vi "Teleop.vi"(10 "Match Info":T1={"Autonomous Elapsed Seconds"=0.0, "TeleOp Elapsed Seconds"=0.0, "Disabled Elapsed Seconds"=0.0, "Visited Autonomous"=FALSE, "Visited TeleOp"=FALSE, "Visited Disabled"=FALSE, "Autonomous Settings"={"Autonomous Style"=enum."Independent", "VI Refnum"=refnum}}, 11 "Call Context":T2) -> ()   [LabVIEW 2020]
doc: "This VI is called for each enabled TeleOp packet received from the DS. It is typically used to read from joysticks and other inputs and update I/O or setpoints for timed control loops. It should complete and return within 20 milliseconds or risk missing DS packets."
uses:
  <vilib>/Rock Robotics/WPI/DriverStation/WPI_DriverStationDerivedRobotMode.ctl
  <vilib>/Rock Robotics/WPI/DriverStation/WPI_DriverStationMatch Info.ctl
  <vilib>/Rock Robotics/WPI/Utilities/WPI_GetSetVariantRefNum.vi
  <vilib>/Rock Robotics/Network Tables/NT Write Boolean Array.vi
  <vilib>/Rock Robotics/Network Tables/NT Write Numeric Array.vi
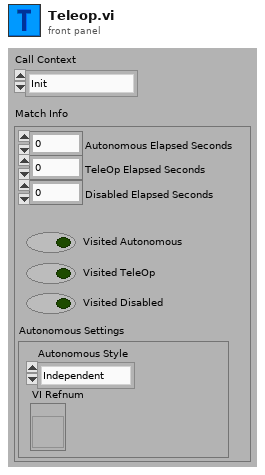
[diagram p1: front panel]
types:
  T1 = typedef "WPI_DriverStationMatch Info.ctl" = cluster{"Autonomous Elapsed Seconds":dbl, "TeleOp Elapsed Seconds":dbl, "Disabled Elapsed Seconds":dbl, "Visited Autonomous":bool, "Visited TeleOp":bool, "Visited Disabled":bool, "Autonomous Settings":cluster{"Autonomous Style":enum16{"Iterative", "Independent"}, "VI Refnum":refnum<vi>}}
  T2 = typedef "WPI_DriverStationDerivedRobotMode.ctl" = enum16{"Init", "Execute", "Stop"}
  T3 = typedef "WPI_JoystickDevRef.ctl" = cluster{"Device":T4}
  T4 = typedef "WPI_JoystickDeviceEnum.ctl" = enum16{"USB 0", "USB 1", "USB 2", "USB 3", "USB 4", "USB 5"}
  T5 = typedef "Command Status Info.ctl" = cluster{"Name":string, "Status":T6, "notifier out":T7}
  T6 = typedef "Completion Status.ctl" = enum16{"Successful", "Aborted", "Incomplete"}
  T7 = typedef "Completion Notifier.ctl" = refnum<notifier>
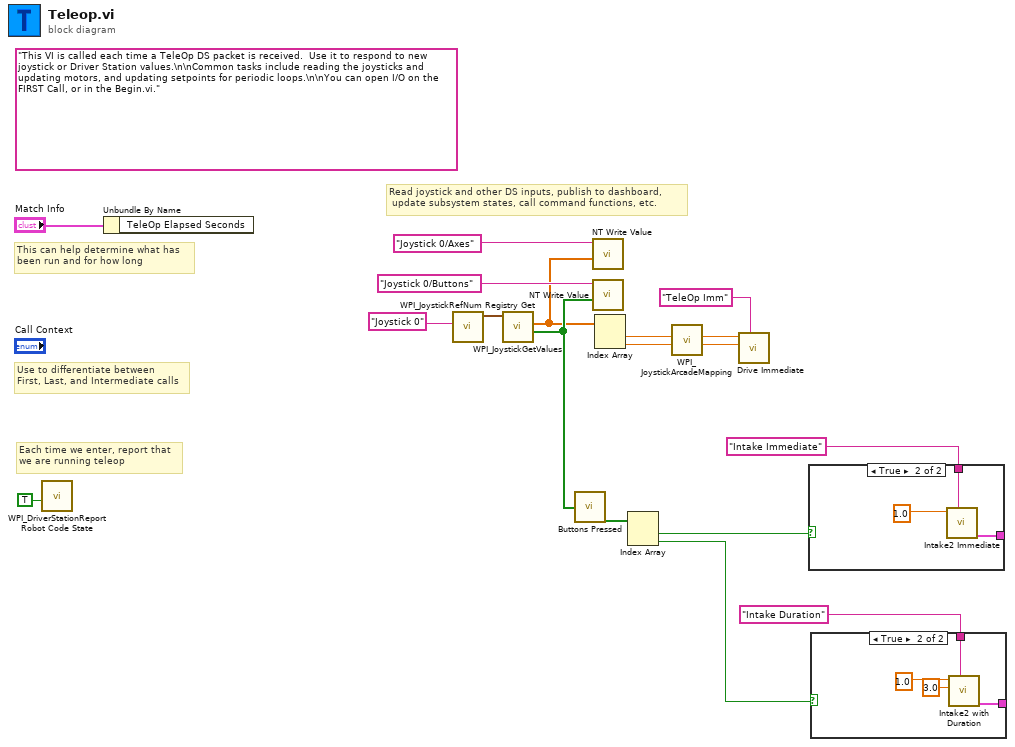
[diagram p0: block diagram]
diagram:
  (unwired) "This VI is called each time a TeleOp DS packet is received.  Use it to respond to new joystick or Driver Station values.\n\nCommon tasks include reading the joysticks and updating motors, and updating setpoints for periodic loops.\n\nYou can open I/O on the FIRST Call, or in the Begin.vi."
  # "Read joystick and other DS inputs, publish to dashboard,\n update subsystem states, call command functions, etc."
  # "Each time we enter, report that\nwe are running teleop"
  # "Use to differentiate between\nFirst, Last, and Intermediate calls"
  # "This can help determine what has\nbeen run and for how long"
  n1 = call <vilib>:"WPI_DriverStationReport Robot Code State.vi"("TeleOp"=TRUE ("Autonomous")) -> ()  [unwired: 10 in, 1 out]
  n2 = Unbundle By Name("Match Info") -> ()  [unwired: 1 out]
  n3 = call <vilib>:"WPI_JoystickRefNum Registry Get.vi"("refnum name"="Joystick 0") -> ("JoystickDevRef"=w15:T3)  [unwired: 1 in, 9 out]
  n4 = call <vilib>:"WPI_JoystickGetValues.vi"("JoystickDevRef"=w15) -> ("Buttons"=w5:bool[], "Axes"=w4:dbl[])  [unwired: 6 in, 3 out]
  n5 = call "Buttons Pressed.vi"("Button Values"=w5) -> ("Button Presses"=w12:bool[])
  n6 = call-poly <vilib>:"NT Write Value.vi"("Numeric Array"=w4, "Name"="Joystick 0/Axes") -> ()  [unwired: 9 in, 1 out]
  n7 = call-poly <vilib>:"NT Write Value.vi"("Boolean Array"=w5, "Name"="Joystick 0/Buttons") -> ()  [unwired: 9 in, 1 out]
  n8 = Index Array(array=w4) -> (element #1=w8:dbl, element #2=w7:dbl)  [unwired: 2 in]
  n9 = Index Array(array=w12) -> (element #1=w11:bool, element #2=w1:bool)  [unwired: 2 in]
  n10 = call <vilib>:"WPI_JoystickArcadeMapping.vi"("Y axis value"=w7, "X axis value"=w8) -> ("Right Motor Value"=w9:dbl, "Left Motor Value"=w10:dbl)  [unwired: 8 in]
  n11 = call "Drive Immediate.vi"("Description"="TeleOp Imm", "Right Setpoint"=w9, "Left Setpoint"=w10) -> ()  [unwired: 8 in, 1 out]
  n12 = case shown="True" w11 {
    tunnel: [_ w21] -> _
    tunnel: "Intake Immediate" ("Description") -> [_ w20]
    frame False {
    }
    frame True {
      n13 = call "Intake2 Immediate.vi"("Description"=w20, "Setpoint"=1.0) -> ("Command Info Out"=w21:T5)  [unwired: 9 in]
    }
  }
  n14 = case shown="True" w1 {
    tunnel: [_ w25] -> _
    tunnel: "Intake Duration" ("Description") -> [_ w24]
    frame False {
    }
    frame True {
      n15 = call "Intake2 with Duration.vi"("Description"=w24, "Duration (s)"=3.0, "Setpoint"=1.0) -> ("Command Info Out"=w25:T5)  [unwired: 8 in]
    }
  }
